vi "TEMPDo.vi"(8 "error in (no error)":errorcluster, 10 "Actor in":refnum<class "Actor.lvclass">, 11 "DNL_Message Template":refnum<class "Message.lvclass">) -> (0 "error out":errorcluster, 2 "Actor out":refnum<class "Actor.lvclass">)   [LabVIEW 2016, in "AsynchReturnDialog Template.lvclass"]
doc: "This VI delivers the message to the actor by calling the appropriate method(s) on the actor."
uses:
  AsynchReturnDialog Template.lvclass
  <vilib>/ActorFramework/Actor/Actor.lvclass
  <vilib>/ActorFramework/Message/Message.lvclass
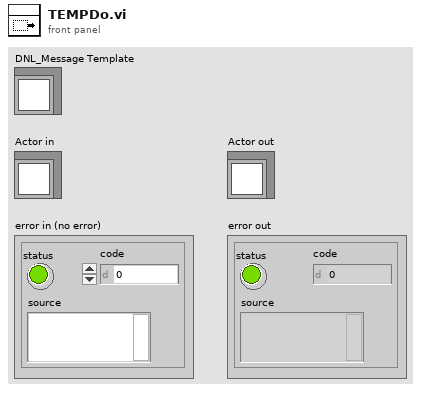
[diagram p1: front panel]
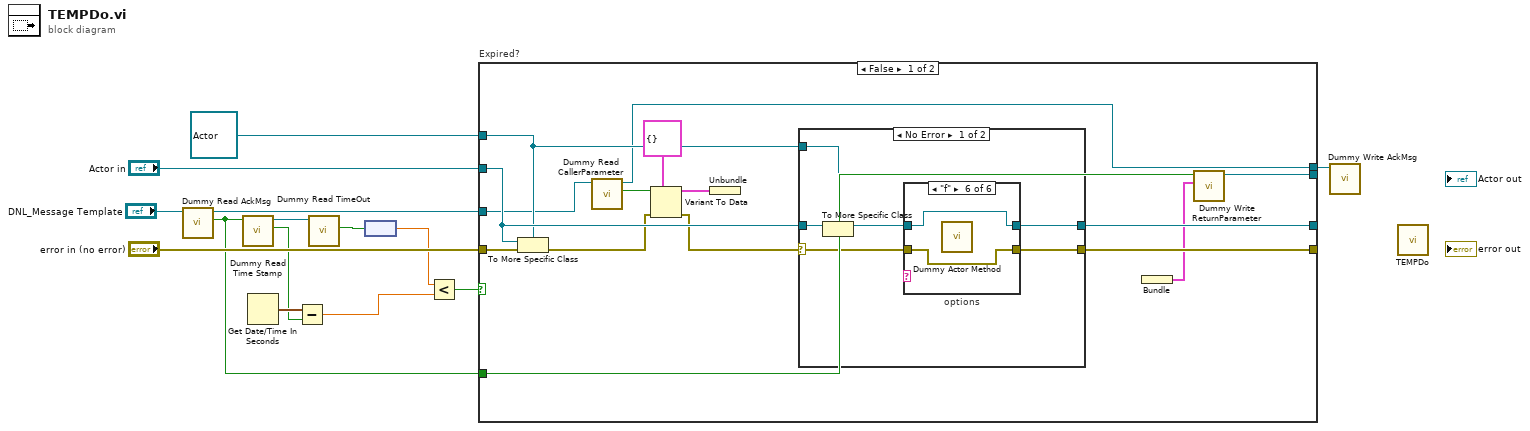
[diagram p0: block diagram]
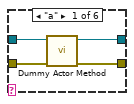
[diagram p2: hidden frame]
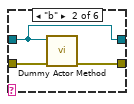
[diagram p3: hidden frame]
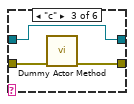
[diagram p4: hidden frame]
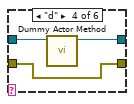
[diagram p5: hidden frame]
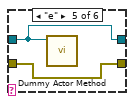
[diagram p6: hidden frame]
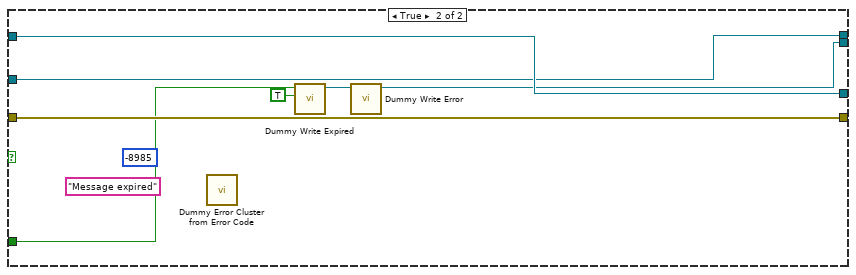
[diagram p8: hidden frame]
diagram:
  n1 = call "Dummy Read AckMsg.vi"("Actor in"="DNL_Message Template") -> ("Boolean"=w2:bool, "Actor out"=w3:refnum<class "Actor.lvclass">)  [unwired: 8 in, 1 out]
  n2 = call "Dummy Read Time Stamp.vi"("Actor in"=w2) -> ("Boolean"=w9:bool, "Actor out"=w8:refnum<class "Actor.lvclass">)  [unwired: 8 in, 1 out]
  n3 = Get Date/Time In Seconds() -> (seconds since 1Jan1904=w10:timestamp)
  n4 = Subtract(x=w10, y=w9) -> (x-y=w5:dbl)
  n5 = call "Dummy Read TimeOut.vi"("Actor in"=w8) -> ("Boolean"=w7:bool)  [unwired: 8 in, 2 out]
  n6 = node(w7) -> (w6:dbl[unit])
  n7 = Less?(x=w6, y=w5) -> (x < y?=w4:bool)
  n8 = case "Expired?" shown="False" w4 {
    tunnel: [w29 w60] -> _
    tunnel: [w28 w61] -> _
    tunnel: "Actor in" -> [w27 w61]
    tunnel: refnum<class "Actor.lvclass"> refnum ("Actor in") -> [w26 _]
    tunnel: "error in (no error)" -> [w25 w60]
    tunnel: w3 -> [w22 w56]
    tunnel: [w18 w56] -> w1
    tunnel: w2 -> [w19 w57]
    tunnel: [w17 w55] -> _
    frame False {
      n9 = To More Specific Class(target class=w26, reference=w27, error in=w25) -> (error out=w16:errorcluster)  [unwired: 1 out]
      n10 = call "Dummy Read CallerParameter.vi"("Actor in"=w22) -> ("Boolean"=w21:bool, "Actor out"=w18:refnum<class "Actor.lvclass">)  [unwired: 8 in, 1 out]
      n11 = Variant To Data(error in=w16, type=cluster{} {} ("Type"), Variant=w21) -> (data=w23:cluster{}, error out=w15:errorcluster)
      n12 = Unbundle ("Main-Unbundler")(w23) -> ()  [unwired: 1 out]
      n13 = case "Error Case" shown="No Error" w15 {
        selector: w15 -> [w33 w54]
        tunnel: [w35 w54] -> w29
        tunnel: [w34 w53] -> w28
        tunnel: w27 -> [w32 w53]
        tunnel: w26 -> [w31 _]
        frame No Error {
          n14 = To More Specific Class(target class=w31, reference=w32) -> (specific class reference=w30:refnum<class "Actor.lvclass">)  [unwired: 1 in, 1 out]
          n15 = case "options" shown="\"f\"" {
            selector: _ -> [_ _ _ _ _ _]
            tunnel: [w39 w42 w45 w48 w49 w51] -> w35
            tunnel: [w38 w40 w43 w46 w50 w52] -> w34
            tunnel: w33 -> [w37 w41 w44 w48 w49 w51]
            tunnel: w30 -> [w36 w40 w43 w47 w50 w52]
            frame "a" {
              n16 = call "Dummy Actor Method.vi"("error in (no error)"=w37, "Actor in"=w36) -> ("error out"=w39:errorcluster, "Actor out"=w38:refnum<class "Actor.lvclass">)  [unwired: 8 in]
            }
            frame "b" {
              n17 = call "Dummy Actor Method.vi"("error in (no error)"=w41, "Actor in"=w40) -> ("error out"=w42:errorcluster)  [unwired: 8 in, 1 out]
            }
            frame "c" {
              n18 = call "Dummy Actor Method.vi"("error in (no error)"=w44) -> ("error out"=w45:errorcluster)  [unwired: 9 in, 1 out]
            }
            frame "d" {
              n19 = call "Dummy Actor Method.vi"("Actor in"=w47) -> ("Actor out"=w46:refnum<class "Actor.lvclass">)  [unwired: 9 in, 1 out]
            }
            frame "e" {
              n20 = call "Dummy Actor Method.vi"("Actor in"=w50) -> ()  [unwired: 9 in, 2 out]
            }
            frame "f" {
              n21 = call "Dummy Actor Method.vi"() -> ()  [unwired: 10 in, 2 out]
            }
          }
        }
        frame Error {
        }
      }
      n22 = Bundle ("Out-Bundler")() -> (w20:cluster{void})  [unwired: 2 in]
      n23 = call "Dummy Write ReturnParameter.vi"("Boolean"=w20, "Actor in"=w19) -> ("Actor out"=w17:refnum<class "Actor.lvclass">)  [unwired: 7 in, 1 out]
    }
    frame True {
      (unwired) -8985 ("ErrorCode")
      (unwired) "Message expired" ("ErrorMsg")
      n24 = call "Dummy Error Cluster from Error Code.vi"() -> ()  [unwired: 9 in, 3 out]
      n25 = call "Dummy Write Expired.vi"("Boolean"=TRUE, "Actor in"=w57) -> ("Actor out"=w59:refnum<class "Actor.lvclass">)  [unwired: 7 in, 1 out]
      n26 = call "Dummy Write Error.vi"("Actor in"=w59) -> ("Actor out"=w55:refnum<class "Actor.lvclass">)  [unwired: 8 in, 1 out]
    }
  }
  n27 = call "Dummy Write AckMsg.vi"("Actor in"=w1) -> ()  [unwired: 9 in, 2 out]
  n28 = call-parent "TEMPDo.vi"() -> ()  [unwired: 1 in]
